vi "Boiler Controller.vi"(8 "error in":errorcluster, 11 "Message Queues":T1) -> (0 "error out":errorcluster)   [LabVIEW 2022 SP3]
uses:
  support/Message Queue/All Message Queues.ctl
  support/Message Queue/Message Cluster.ctl
  support/Message Queue/Message Queue.lvlib
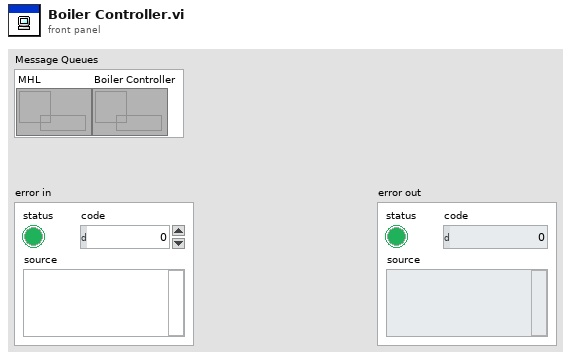
[diagram p1: front panel]
types:
  T1 = typedef "Message Queue.lvlib/All Message Queues.ctl" = cluster{"MHL":refnum<queue>, "Boiler Controller":refnum<queue>}
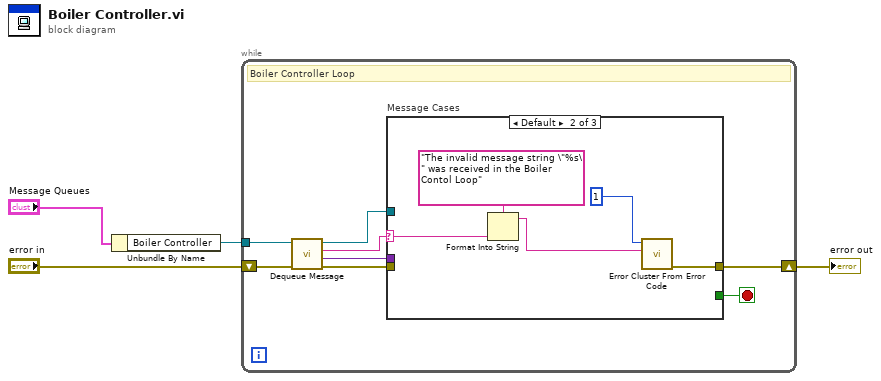
[diagram p0: block diagram]
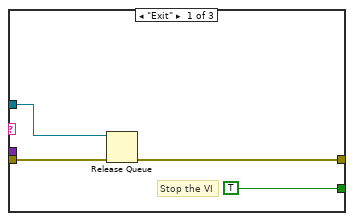
[diagram p2: hidden frame]
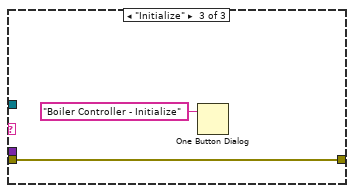
[diagram p3: hidden frame]
diagram:
  n1 = Unbundle By Name("Message Queues") -> ("Boiler Controller"=w3:refnum<queue>)
  n2 = while {
    tunnel: w3 -> [w12]
    shift-right: [w6] -> w1
    shift-left: "error in" -> [w7]
    stop <- w5 stop-if-true
    # "Boiler Controller Loop"
    n3 = call "Dequeue Message.vi"("error in"=w7, "Message Queue"=w12) -> ("error out"=w8:errorcluster, "Message Data"=w9:variant, "Message"=w11:string, "dup Message Queue"=w10:refnum<queue>)  [unwired: 6 in]
    n4 = case "Message Cases" shown="Default" w11 {
      selector: w11 -> [_ w21 _]
      tunnel: w10 -> [w16 _ _]
      tunnel: w9 -> [_ _ _]
      tunnel: w8 -> [w15 _ w22]
      tunnel: [w14 w19 w22] -> w6
      tunnel: [TRUE _ _] -> w5
      frame "Exit" {
        # "Stop the VI"
        n5 = Release Queue(queue=w16, error in (no error)=w15) -> (error out=w14:errorcluster)  [unwired: 1 in, 2 out]
      }
      frame Default {
        n6 = Format Into String(format string="The invalid message string \"%s\" was received in the Boiler Contol Loop", w21) -> (resulting string=w18:string)  [unwired: 2 in, 1 out]
        n7 = call <vilib>:"Error Cluster From Error Code.vi"("error message (\"\")"=w18, "error code (0)"=1) -> ("error out"=w19:errorcluster)  [unwired: 7 in]
      }
      frame "Initialize" {
        n8 = One Button Dialog(message="Boiler Controller - Initialize") -> ()  [unwired: 1 in, 1 out]
      }
    }
  }
  "error out" <- w1
